vi "IsOpen.vi"() -> ()   [LabVIEW 2017]
panel:
  out "x != y?":bool
  out "standard output":string
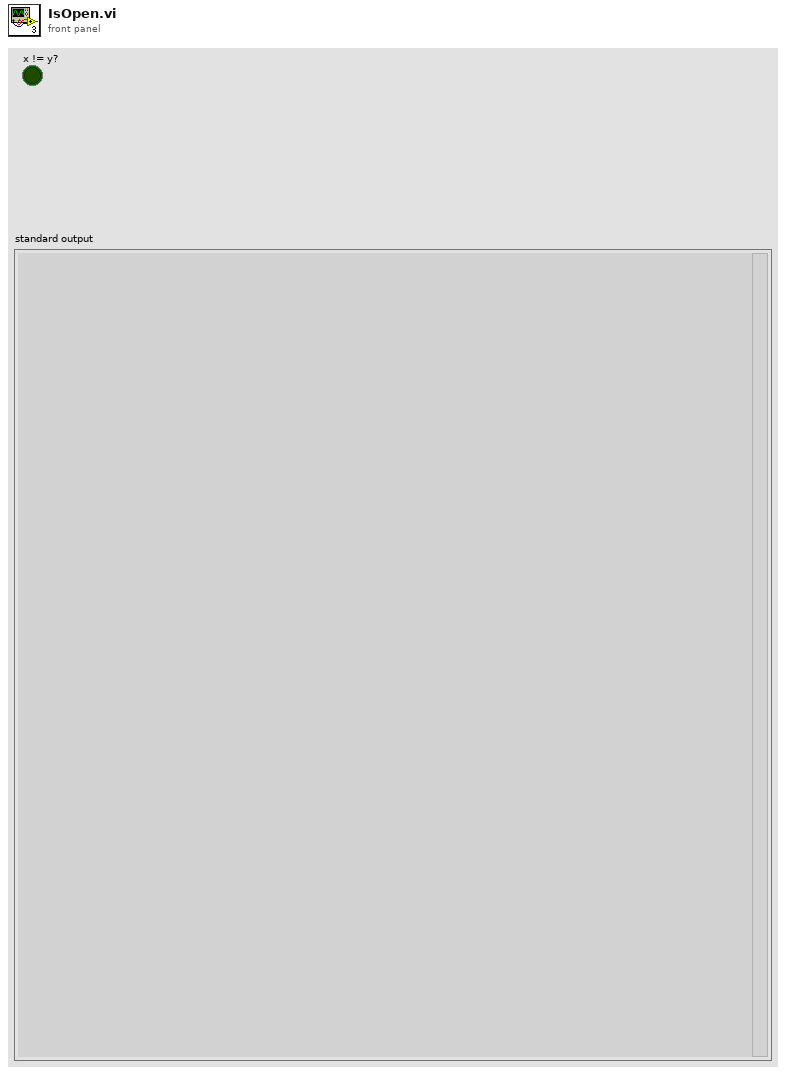
[diagram p1: front panel]
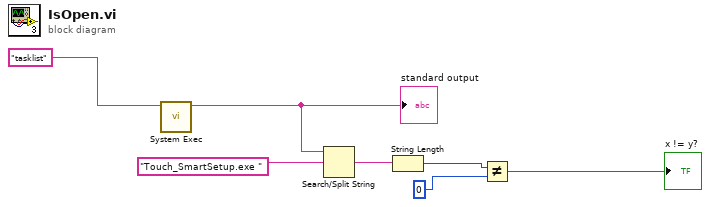
[diagram p0: block diagram]
diagram:
  n1 = call <vilib>:"System Exec.vi"("command line"="tasklist") -> ("standard output"=w6:string)  [unwired: 7 in, 3 out]
  "standard output" <- w6
  n2 = Search/Split String(string=w6, search string/char (-)="Touch_SmartSetup.exe ") -> (match + rest of string=w4:string)  [unwired: 1 in, 2 out]
  n3 = String Length(string=w4) -> (length=w3:i32)
  n4 = Not Equal?(x=w3, y=0) -> (x != y?=→"x != y?":bool)
